vi "subPropertyGetTagValue.vi"(8 "error in (no error)":errorcluster, 10 "Tag Name":string, 11 "ProjectItem in":refnum<vi>) -> (3 "Value":string)   [LabVIEW 2020, in "SolutionBuilder.lvlib"]
uses:
  SolutionBuilder.lvlib
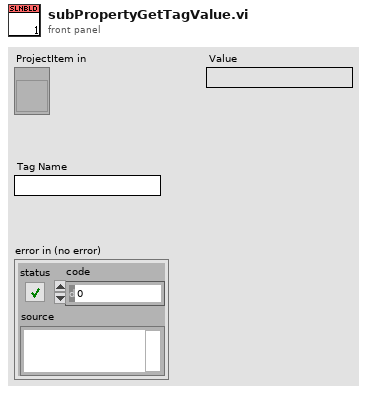
[diagram p1: front panel]
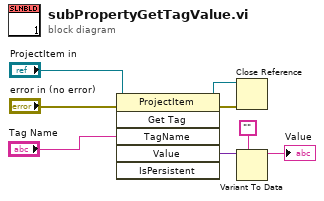
[diagram p0: block diagram]
diagram:
  n1 = invoke class="ProjectItem" method="Get Tag"(reference="ProjectItem in", error in="error in (no error)", "TagName"="Tag Name") -> (reference out=w8:refnum<vi>, error out=w7:errorcluster, "Value"=w4:variant)  [unwired: 3 in, 3 out]
  n2 = Close Reference(reference=w8, error in (no error)=w7) -> ()  [unwired: 1 out]
  n3 = Variant To Data(type="", Variant=w4) -> (data=→"Value":string)  [unwired: 1 in, 1 out]
